vi "CVT Enum Read.vi"(3 "error in (no error)":errorcluster, 5 "Tag Name":string) -> (0 "error out":errorcluster, 1 "Value":i32)   [LabVIEW 2020, in "Current Value Table(Rebuild).lvlib"]
uses:
  _SubVIs/TypeDefs/cvt_MemBlock Methods.ctl
  _SubVIs/TypeDefs/cvt_TagList Methods.ctl
  Current Value Table(Rebuild).lvlib
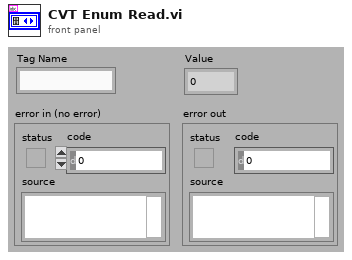
[diagram p1: front panel]
types:
  T1 = typedef "Current Value Table(Rebuild).lvlib/cvt_MemBlock Methods.ctl" = enum16{"init", "read", "readall", "write"}
  T2 = typedef "Current Value Table(Rebuild).lvlib/cvt_TagList Methods.ctl" = enum16{"init", "getindex", "getdesc", "getlist"}
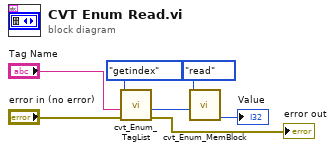
[diagram p0: block diagram]
diagram:
  n1 = call "cvt_Enum_TagList.vi"("error in (no error)"="error in (no error)", "Tag Name"="Tag Name", "Method"=cvt_TagList_Methods."getindex") -> ("error out"=→"error out":errorcluster, "Index"=w6:i32)  [unwired: 1 in, 6 out]
  n2 = call "cvt_Enum_MemBlock.vi"("Index"=w6, "Method"=cvt_MemBlock_Methods."read") -> ("Value"=→"Value":i32)  [unwired: 2 in, 7 out]
